vi "HFRR ADV v07 new software.vi"() -> ()   [LabVIEW 2025] (continued)
              n1275 = local write "Language Selection"(w1589) -> ()
            }
            frame 11 {
              n1276 = local write "CH-POWER +"(w1590) -> ()
            }
            frame 12 {
              n1277 = local write "CH-POWER -"(w1591) -> ()
            }
            frame 13 {
              n1278 = local write "CH-HEATER"(w1592) -> ()
            }
            frame 14 {
              n1279 = local write "CH-HUMIDITY WET"(w1593) -> ()
            }
            frame 15 {
              n1280 = local write "CH-HUMIDITY DRY"(w1594) -> ()
            }
            frame 16 {
            }
            frame 17 {
              n1281 = local write "AIR TEMP INTERCEPT:"(w1595) -> ()
            }
            frame 18 {
              n1282 = local write "TEMP INTERCEPT:"(w1596) -> ()
            }
            frame 21 {
              n1283 = local write "S.NO"(w1597) -> ()
            }
            frame 22 {
              n1284 = local write "Com Port 3"(w1598) -> ()
            }
            frame 20 {
              n1285 = local write "Camera Port :"(w1599) -> ()
            }
            frame 19 {
              n1286 = local write "C3 :"(w1600) -> ()
            }
            frame 23, Default {
            }
          }
        }
      }
    }
    n1287 = Select(t=u32 2500 ("milliseconds to wait"), s=w1553, f=u32 500 ("milliseconds to wait")) -> (s? t:f=w1551:u32)
    n1288 = Multiply(x=w1556, y=w1551) -> (x*y=w1558:dbl)
    n1289 = property on="Time slide" class="Slide (strict)"("Visible"=w1547) -> ()  [unwired: 2 in, 2 out]
    n1290 = call "Elapsed Time2"("Time Target (s)"=w1558, "Auto Reset"=TRUE) -> ("Time has Elapsed"=w1548:bool)  [unwired: 10 in, 7 out]
    n1291 = case shown="True" w1548 {
      frame False {
      }
      frame True {
        n1292 = stacked-sequence {
          frame #0 {
            # "DATA PROCESSING"
            # "115 mV/N"
            n1293 = local read "Sample Temperature"() -> (w1601:dbl)
            "TEMP 2" <- w1601
            "TEMP 3" <- w1601
            n1294 = local read "RH Numeric:"() -> (w1608:dbl)
            n1295 = local read "HUMIDITY:"() -> (w1609:dbl)
            n1296 = local read "FRICVALZ"() -> (w1620:dbl)
            n1297 = local read "Friction"() -> (w1604:dbl)
            n1298 = local write "TEMP"(w1601) -> ()
            n1299 = Multiply(x=w1608, y=w1609) -> (x*y=→"Humidity ( %RH )" →"Hum" →"Hum 2":dbl)
            n1300 = Subtract(x=w1604, y=w1620) -> (x-y=w1615:dbl)
            "FF 2" <- w1615
            "FF 4" <- w1615
            n1301 = local read "Ambient Temperature"() -> (→"AIR TEMP":dbl)
            n1302 = local read "TEMP"() -> (w1619:dbl)
            n1303 = local write "FF 3"(w1615) -> ()
            n1304 = Compound Arithmetic op=OR("FRICVALZ 4", "FRICVALZ 3", "FRICVALZ 2") -> (w1611:bool)
            n1305 = case shown="True" w1611 {
              tunnel: w1604 -> [_ w1626]
              frame False {
              }
              frame True {
                w1625 = FALSE ("FRICVALZ")
                n1306 = local write "FRICVALZ 3"(w1625) -> ()
                n1307 = local write "FRICVALZ 2"(w1625) -> ()
                n1308 = local write "FRICVALZ 4"(w1625) -> ()
                "FRICVALZ" <- w1626
              }
            }
            n1309 = Not A Number/Path/Refnum?(number/path/refnum=w1619) -> (NaN/Path/Refnum?=w1618:bool)
            n1310 = Not A Number/Path/Refnum?(number/path/refnum=w1615) -> (NaN/Path/Refnum?=w1617:bool)
            n1311 = Divide(x=w1615, y=1.96) -> (x/y=w1612:dbl)
            n1312 = Compound Arithmetic op=OR(w1618, w1617) -> (w1616:bool)
            n1313 = Not A Number/Path/Refnum?(number/path/refnum=w1612) -> (NaN/Path/Refnum?=w1613:bool)
            n1314 = case shown="True" w1616 {
              frame False {
              }
              frame True {
                n1315 = local write "TEMP"(0.0 ("TEMP")) -> ()
                n1316 = local write "FF 2"(0.0 ("FF 2")) -> ()
                n1317 = local write "reinit"(TRUE ("reinit")) -> ()
              }
            }
            n1318 = Select(t=0.0, s=w1613, f=w1612) -> (s? t:f=w1603:dbl)
            "COF 2" <- w1603
            n1319 = local write "COF 3"(w1603) -> ()
          }
        }
      }
    }
    n1320 = Wait (ms)(milliseconds to wait=u32 50) -> ()  [unwired: 1 out]
    n1321 = local read "Quit"() -> (w1540:bool)
    "Rate" <- 2500.0 ("No of Samples")
  }
  n1322 = while {
    tunnel: w57 -> [_]
    tunnel: [w1653] -> _
    tunnel: [w1629] -> w56
    i -> [w1653]
    stop <- w1629 stop-if-true
    # "C:\\LAB-IQ-NXT\\Scar View.exe"
    n1323 = local read "OK Button 16"() -> (w1642:bool)
    n1324 = local read "Main Tab"() -> (w1635:T2)
    n1325 = local read "service 3"() -> (w1636:bool)
    n1326 = local read "OPEN 6"() -> (w1638:bool)
    n1327 = local read "EDIT 2"() -> (w1640:bool)
    n1328 = flat-sequence {
      frame #0 {
        n1329 = local read "SAVE 2"() -> (w2255:bool)
        n1330 = stacked-sequence {
          frame #0 {
            n1331 = local read "EDIT"() -> (w2309:bool)
            n1332 = case shown="True" w2309 {
              tunnel: [u8 2 ("Disabled") u8 0 ("Disabled")] -> _
              frame False {
                w2311 = FALSE
                n1333 = local write "Password"("") -> ()
                n1334 = property on="SrvM CP" class="Bool (strict)"("Visible"=w2311) -> ()  [unwired: 2 in, 2 out]
                n1335 = property on="message" class="Str"("Visible"=w2311) -> ()  [unwired: 2 in, 2 out]
                n1336 = local write "x = y?"(w2311) -> ()
                n1337 = property on="Password" class="Str"("Visible"=w2311) -> ()  [unwired: 2 in, 2 out]
                n1338 = property on="ENTER THE NEW PASSWORD" class="Str"("Visible"=w2311) -> ()  [unwired: 2 in, 2 out]
                n1339 = property on="ENTER CURRENT PASSWORD" class="Str"("Visible"=w2311) -> ()  [unwired: 2 in, 2 out]
                n1340 = local write "SrvM CP"(w2311) -> ()
              }
              frame True {
                w2314 = TRUE
                n1341 = property on="SrvM CP" class="Bool (strict)"("Visible"=w2314) -> ()  [unwired: 2 in, 2 out]
                n1342 = property on="Password" class="Str"("Visible"=w2314) -> ()  [unwired: 2 in, 2 out]
              }
            }
            "dipl pwd" <- "@143$\n" ("dipl pwd")
          }
          frame #1 {
            # "Gain password"
            n1343 = String To Byte Array(string="ENTER CURRENT PASSWORD") -> (unsigned byte array=w2319:u8[])
            n1344 = Search 1D Array(1D array=w2319, element=u8 10) -> (index of element=w2322:i32)  [unwired: 1 in]
            n1345 = Index Array(array=w2319, index=w2322) -> (element=w2318:u8)
            n1346 = Equal?(x=w2318, y=10) -> (x = y?=w2316:bool)
            n1347 = case shown="True" w2316 {
              frame False {
                n1348 = property on="ENTER THE NEW PASSWORD" class="Str"("Visible"=FALSE) -> ()  [unwired: 2 in, 2 out]
              }
              frame True {
                # "password"
                # "change password logic"
                n1349 = local read "ENTER CURRENT PASSWORD"() -> (w2335:string)
                n1350 = local read "dipl pwd"() -> (w2329:string)
                n1351 = String To Byte Array(string=w2335) -> (unsigned byte array=w2337:u8[])
                n1352 = String To Byte Array(string=w2329) -> (unsigned byte array=w2330:u8[])
                n1353 = Array Size(array=w2337) -> (size(s)=w2334:i32)
                n1354 = Array Size(array=w2330) -> (size(s)=w2332:i32)
                n1355 = for {
                  N: w2334 -> [_]
                  tunnel: w2337 -> [w2361]
                  tunnel: [w2359] -> w2338 mode=indexing
                  tunnel: w2334 -> [w2353]
                  i -> [w2354]
                  n1356 = Decrement(x=w2353) -> (x-1=w2351:i32)
                  n1357 = Equal?(x=w2354, y=w2351) -> (x = y?=w2352:bool)
                  n1358 = Index Array(array=w2361, index=w2354) -> (element=w2355:u8)
                  n1359 = Number To Decimal String(number=w2355) -> (decimal integer string=w2360:string)  [unwired: 1 in]
                  n1360 = Select(t="", s=w2352, f="\r") -> (s? t:f=w2357:string)
                  n1361 = Concatenate Strings(w2360, w2357) -> (w2359:string)
                }
                n1362 = for {
                  N: w2332 -> [_]
                  tunnel: w2330 -> [w2349]
                  tunnel: [w2347] -> w2331 mode=indexing
                  tunnel: w2332 -> [w2344]
                  i -> [w2345]
                  n1363 = Decrement(x=w2344) -> (x-1=w2343:i32)
                  n1364 = Equal?(x=w2345, y=w2343) -> (x = y?=w2342:bool)
                  n1365 = Index Array(array=w2349, index=w2345) -> (element=w2348:u8)
                  n1366 = Number To Decimal String(number=w2348) -> (decimal integer string=w2346:string)  [unwired: 1 in]
                  n1367 = Select(t="", s=w2342, f="\r") -> (s? t:f=w2339:string)
                  n1368 = Concatenate Strings(w2346, w2339) -> (w2347:string)
                }
                n1369 = local read "string"() -> (w2336:string)
                n1370 = Concatenate Strings(w2331) -> (w2325:string)
                n1371 = Concatenate Strings(w2336) -> (w2333:string)
                n1372 = Concatenate Strings(w2338) -> (w2326:string)
                n1373 = Equal?(x=w2326, y=w2333) -> (x = y?=w2328:bool)
                n1374 = Equal?(x=w2326, y=w2325) -> (x = y?=w2324:bool)
                n1375 = Or(x=w2328, y=w2324) -> (x .or. y?=w2327:bool)
                n1376 = case shown="True" w2327 {
                  frame False {
                  }
                  frame True {
                    n1377 = property on="ENTER THE NEW PASSWORD" class="Str"("Visible"=TRUE) -> ()  [unwired: 2 in, 2 out]
                  }
                }
              }
            }
          }
          frame #2 {
            n1378 = String To Byte Array(string="ENTER THE NEW PASSWORD") -> (unsigned byte array=w2364:u8[])
            n1379 = Search 1D Array(1D array=w2364, element=u8 10) -> (index of element=w2368:i32)  [unwired: 1 in]
            n1380 = Index Array(array=w2364, index=w2368) -> (element=w2366:u8)
            n1381 = Equal?(x=w2366, y=10) -> (x = y?=w2363:bool)
            n1382 = case shown="False" w2363 {
              frame False {
              }
              frame True {
                n1383 = local write "EDIT"(FALSE) -> ()
                n1384 = local write "SrvM CP"(FALSE) -> ()
                n1385 = local read "ENTER THE NEW PASSWORD"() -> (w2371:string)
                n1386 = String To Byte Array(string=w2371) -> (unsigned byte array=w2376:u8[])
                n1387 = Array Size(array=w2376) -> (size(s)=w2373:i32)
                n1388 = for {
                  N: w2373 -> [_]
                  tunnel: w2376 -> [w2389]
                  tunnel: [w2386] -> w2378 mode=indexing
                  tunnel: w2373 -> [w2381]
                  i -> [w2379]
                  n1389 = Decrement(x=w2381) -> (x-1=w2382:i32)
                  n1390 = Equal?(x=w2379, y=w2382) -> (x = y?=w2383:bool)
                  n1391 = Index Array(array=w2389, index=w2379) -> (element=w2388:u8)
                  n1392 = Number To Decimal String(number=w2388) -> (decimal integer string=w2387:string)  [unwired: 1 in]
                  n1393 = Select(t="", s=w2383, f="\r") -> (s? t:f=w2380:string)
                  n1394 = Concatenate Strings(w2387, w2380) -> (w2386:string)
                }
                n1395 = local read "file path"() -> (w2370:path)
                n1396 = Concatenate Strings(w2378) -> (w2372:string)
                n1397 = Delete(path (use dialog)=w2370) -> (deleted path=w2374:path)  [unwired: 4 in, 2 out]
                n1398 = call <vilib>:"Write Characters To File.vi"("append to file? (new file:F)"=FALSE, "character string"=w2372, "file path (dialog if empty)"=w2374) -> ()  [unwired: 2 in, 1 out]
              }
            }
          }
          frame #3 {
            n1399 = case shown="True" "SrvM CP" {
              frame False {
                w2392 = ""
                n1400 = local write "ENTER CURRENT PASSWORD"(w2392) -> ()
                n1401 = local write "ENTER THE NEW PASSWORD"(w2392) -> ()
                n1402 = property on="ENTER CURRENT PASSWORD" class="Str"("Visible"=FALSE) -> ()  [unwired: 2 in, 2 out]
              }
              frame True {
                n1403 = property on="ENTER THE NEW PASSWORD" class="Str"() -> ("Visible"=w2393:bool)  [unwired: 2 in, 2 out]
                n1404 = Not(x=w2393) -> (.not. x?=w2394:bool)
                n1405 = property on="ENTER CURRENT PASSWORD" class="Str"("Visible"=w2394) -> ()  [unwired: 2 in, 2 out]
              }
            }
          }
          frame #4 {
            n1406 = String To Byte Array(string="Password") -> (unsigned byte array=w2401:u8[])
            n1407 = Search 1D Array(1D array=w2401, element=u8 10) -> (index of element=w2399:i32)  [unwired: 1 in]
            n1408 = Index Array(array=w2401, index=w2399) -> (element=w2400:u8)
            n1409 = Equal?(x=w2400, y=10) -> (x = y?=w2396:bool)
            n1410 = case shown="True" w2396 {
              frame False {
              }
              frame True {
                # "password"
                # "password"
                n1411 = local read "Password"() -> (w2414:string)
                n1412 = String To Byte Array(string=w2414) -> (unsigned byte array=w2417:u8[])
                n1413 = String To Byte Array(string="@143$\n") -> (unsigned byte array=w2403:u8[])
                n1414 = Array Size(array=w2417) -> (size(s)=w2412:i32)
                n1415 = Array Size(array=w2403) -> (size(s)=w2408:i32)
                n1416 = for {
                  N: w2412 -> [_]
                  tunnel: w2417 -> [w2451]
                  tunnel: [w2449] -> w2418 mode=indexing
                  tunnel: w2412 -> [w2446]
                  i -> [w2447]
                  n1417 = Decrement(x=w2446) -> (x-1=w2445:i32)
                  n1418 = Index Array(array=w2451, index=w2447) -> (element=w2450:u8)
                  n1419 = Equal?(x=w2447, y=w2445) -> (x = y?=w2444:bool)
                  n1420 = Number To Decimal String(number=w2450) -> (decimal integer string=w2448:string)  [unwired: 1 in]
                  n1421 = Select(t="", s=w2444, f="\r") -> (s? t:f=w2441:string)
                  n1422 = Concatenate Strings(w2448, w2441) -> (w2449:string)
                }
                n1423 = for {
                  N: w2408 -> [_]
                  tunnel: w2403 -> [w2462]
                  tunnel: [w2460] -> w2406 mode=indexing
                  tunnel: w2408 -> [w2457]
                  i -> [w2458]
                  n1424 = Decrement(x=w2457) -> (x-1=w2456:i32)
                  n1425 = Index Array(array=w2462, index=w2458) -> (element=w2461:u8)
                  n1426 = Equal?(x=w2458, y=w2456) -> (x = y?=w2455:bool)
                  n1427 = Number To Decimal String(number=w2461) -> (decimal integer string=w2459:string)  [unwired: 1 in]
                  n1428 = Select(t="", s=w2455, f="\r") -> (s? t:f=w2452:string)
                  n1429 = Concatenate Strings(w2459, w2452) -> (w2460:string)
                }
                n1430 = local read "file path"() -> (w2402:path)
                n1431 = call <vilib>:"Read Characters From File.vi"("file path (dialog if empty)"=w2402) -> ("character string"=w2416:string)  [unwired: 5 in, 3 out]
                "string" <- w2416
                n1432 = flat-sequence {
                  tunnel: [w2419] -> w2413
                  frame #0 {
                    w2419 = ""
                    n1433 = local write "Password"(w2419) -> ()
                  }
                }
                n1434 = Concatenate Strings(w2406) -> (w2407:string)
                n1435 = Concatenate Strings(w2416) -> (w2415:string)
                n1436 = Concatenate Strings(w2418) -> (w2410:string)
                n1437 = Equal?(x=w2410, y=w2415) -> (x = y?=w2405:bool)
                n1438 = Equal?(x=w2410, y=w2407) -> (x = y?=w2411:bool)
                n1439 = Or(x=w2405, y=w2411) -> (x .or. y?=w2404:bool)
                "x = y?" <- w2404
                n1440 = case shown="True" w2404 {
                  selector: w2404 -> [w2421 _]
                  tunnel: w2413 -> [_ _]
                  frame False {
                    n1441 = And(x=w2421, y=TRUE ("Visible")) -> (x .and. y?=w2422:bool)
                    n1442 = property on="message" class="Str"("Visible"=w2422) -> ()  [unwired: 2 in, 2 out]
                  }
                  frame True {
                    n1443 = control-ref of="This VI"() -> (w2433:refnum<vi>)
                    n1444 = property class="VI"(reference=w2433) -> (reference out=w2424:refnum<vi>, error out=w2428:errorcluster, "Panel"=w2432:refnum<vi>)  [unwired: 1 in]
                    n1445 = property on="message" class="Str"("Visible"=FALSE) -> ()  [unwired: 2 in, 2 out]
                    n1446 = property class="Pnl"(reference=w2432, error in=w2428) -> (reference out=w2426:refnum<vi>, error out=w2429:errorcluster, "Panes[]"=w2431:refnum<vi>[])
                    n1447 = for {
                      tunnel: w2431 -> [w2440] mode=indexing
                      tunnel: T18."Always On" ("Horizontal Scrollbar Visibility") -> [w2439]
                      tunnel: w2429 -> [w2436]
                      tunnel: [w2435] -> w2427
                      n1448 = property class="Pane"(reference=w2440, error in=w2436, "HorizScrollbarVisibility"=w2439) -> (reference out=w2437:refnum<vi>, error out=w2438:errorcluster)
                      n1449 = Close Reference(reference=w2437, error in (no error)=w2438) -> (error out=w2435:errorcluster)
                    }
                    n1450 = Close Reference(reference=w2426, error in (no error)=w2427) -> (error out=w2425:errorcluster)
                    n1451 = Close Reference(reference=w2424, error in (no error)=w2425) -> (error out=→"error out 6":errorcluster)
                  }
                }
              }
            }
          }
        }
        n1452 = local read "x = y?"() -> (w2261:bool)
        n1453 = local read "HUMIDITY: 2"() -> (w2263:dbl)
        n1454 = local read "HUMIDITY:"() -> (w2262:dbl)
        n1455 = property on="Port 2 Error" class="Clust (strict)"("Visible"="EDIT") -> ()  [unwired: 2 in, 2 out]
        n1456 = property on="Port 1 Error" class="Clust (strict)"("Visible"="EDIT") -> ()  [unwired: 2 in, 2 out]
        n1457 = case shown="True" "SrvM CP 2" {
          frame False {
          }
          frame True {
            n1458 = local write "SrvM CP 2"(FALSE ("SrvM CP 2")) -> ()
            n1459 = local read "HUMIDITY: 2"() -> (w2302:dbl)
            n1460 = local read "TEMP INTERCEPT: 2"() -> (w2301:dbl)
            n1461 = local read "DISPLACEMENT : 4"() -> (w2305:dbl)
            n1462 = local read "TEMPERATURE : 2"() -> (w2304:dbl)
            n1463 = local read "STROKE GAIN : 2"() -> (w2306:dbl)
            n1464 = local read "FRIC. FORCE : 2"() -> (w2307:dbl)
            n1465 = local read "AIR TEMP INTERCEPT: 2"() -> (w2300:dbl)
            n1466 = local read "AIR TEMPERATURE : 2"() -> (w2303:dbl)
            n1467 = local write "HUMIDITY:"(w2302) -> ()
            n1468 = local write "AIR TEMP INTERCEPT:"(w2301) -> ()
            n1469 = local write "TEMPERATURE :"(w2304) -> ()
            n1470 = local write "FRIC. FORCE :"(w2307) -> ()
            n1471 = local write "STROKE GAIN :"(w2306) -> ()
            n1472 = local write "DISPLACEMENT :"(w2305) -> ()
            n1473 = local write "AIR TEMPERATURE :"(w2303) -> ()
            n1474 = local write "TEMP INTERCEPT:"(w2300) -> ()
          }
        }
        n1475 = Or(x="SAVE", y=w2255) -> (x .or. y?=w2256:bool)
        n1476 = And(x="EDIT", y=w2261) -> (x .and. y?=w2259:bool)
        n1477 = local read "DISPLACEMENT : 4"() -> (w2272:dbl)
        n1478 = local read "TEMPERATURE : 2"() -> (w2270:dbl)
        n1479 = local read "STROKE GAIN : 2"() -> (w2276:dbl)
        n1480 = local read "DISPLACEMENT :"() -> (w2271:dbl)
        n1481 = local read "FRIC. FORCE : 2"() -> (w2279:dbl)
        n1482 = local read "TEMPERATURE :"() -> (w2268:dbl)
        n1483 = local read "STROKE GAIN :"() -> (w2275:dbl)
        n1484 = local read "FRIC. FORCE :"() -> (w2278:dbl)
        n1485 = case shown="True" w2259 {
          tunnel: [u8 2 ("Disabled") u8 0 ("Disabled")] -> w2258
          tunnel: [w2623 TRUE ("Visible")] -> w2257
          frame False {
            w2623 = FALSE ("Visible")
            n1486 = local write "EDIT 2"(w2623) -> ()
          }
          frame True {
          }
        }
        n1487 = case shown="True" w2256 {
          frame False {
          }
          frame True {
            n1488 = stacked-sequence {
              seq-local: [w2471 _ _] -> [_ w2618 _]
              frame #0 {
                (unwired) i16 5 ("precision (6)")
                # "[CH1]    - FF\n[CH2]   - TEMPERATURE\n[CH3]    - Humidity\n[CH4]    - AIR TEMP\n[CH5]\\- Visa Uno\n[CH6] \\- Visa Due\n[CH7]  \\- file path\n[CH8]   - Displacement Gain\n[CHA]   - Stroke Gain\n[CHB]   - Stroke PID Gain\n[CHC]   -Language Selection\n[CHD]   -Power +\n[CHE]   -Power_\n[CHF]   -Heater\n[CHG]   -Humidity Wet\n[CHH]   -Humidity Dry\n[CHI]   -Integral Time"
                n1489 = local read "Language Selection"() -> (w2519:enum16{"English", "Russian"})
                n1490 = local read "CH-HUMIDITY WET"() -> (w2477:u16)
                n1491 = local read "CH-HUMIDITY DRY"() -> (w2474:u16)
                n1492 = local read "STROKE GAIN :"() -> (w2463:dbl)
                n1493 = local read "CH-POWER +"() -> (w2486:u16)
                n1494 = local read "CH-POWER -"() -> (w2483:u16)
                n1495 = local read "CH-HEATER"() -> (w2480:u16)
                n1496 = local read "AIR TEMPERATURE :"() -> (w2466:dbl)
                n1497 = local read "DISPLACEMENT :"() -> (w2464:dbl)
                n1498 = local read "TEMPERATURE :"() -> (w2467:dbl)
                n1499 = local read "FRIC. FORCE :"() -> (w2468:dbl)
                n1500 = local read "HUMIDITY:"() -> (w2465:dbl)
                n1501 = Path To String(path="File Path") -> (string=w2535:string)
                n1502 = Number To Fractional String(number=w2463, width (-)=i16 10 ("precision (6)"), precision (6)=i16 5) -> (F-format string=w2526:string)  [unwired: 1 in]
                n1503 = Number To Fractional String(number=w2519, width (-)=i16 10 ("precision (6)"), precision (6)=i16 5) -> (F-format string=w2515:string)  [unwired: 1 in]
                n1504 = Number To Fractional String(number=w2486, width (-)=i16 10 ("precision (6)"), precision (6)=i16 5) -> (F-format string=w2509:string)  [unwired: 1 in]
                n1505 = Number To Fractional String(number=w2483, width (-)=i16 10 ("precision (6)"), precision (6)=i16 5) -> (F-format string=w2506:string)  [unwired: 1 in]
                n1506 = Number To Fractional String(number=w2480, width (-)=i16 10 ("precision (6)"), precision (6)=i16 5) -> (F-format string=w2501:string)  [unwired: 1 in]
                n1507 = Number To Fractional String(number=w2477, width (-)=i16 10 ("precision (6)"), precision (6)=i16 5) -> (F-format string=w2498:string)  [unwired: 1 in]
                n1508 = Number To Fractional String(number=w2474, width (-)=i16 10 ("precision (6)"), precision (6)=i16 5) -> (F-format string=w2493:string)  [unwired: 1 in]
                n1509 = local read "Com Port 1"() -> (w2470:refnum<visa-resource-name>)
                n1510 = local read "Com Port 2"() -> (w2469:refnum<visa-resource-name>)
                n1511 = Concatenate Strings(w2535, "\\" ("string")) -> (w2534:string)
                n1512 = Number To Fractional String(number=w2468, width (-)=i16 10 ("precision (6)"), precision (6)=i16 5) -> (F-format string=w2567:string)  [unwired: 1 in]
                n1513 = Number To Fractional String(number=w2467, width (-)=i16 10 ("precision (6)"), precision (6)=i16 5) -> (F-format string=w2566:string)  [unwired: 1 in]
                n1514 = Number To Fractional String(number=w2465, width (-)=i16 10 ("precision (6)"), precision (6)=i16 5) -> (F-format string=w2560:string)  [unwired: 1 in]
                n1515 = Number To Fractional String(number=w2466, width (-)=i16 10 ("precision (6)"), precision (6)=i16 5) -> (F-format string=w2554:string)  [unwired: 1 in]
                n1516 = Number To Fractional String(number=w2464, width (-)=i16 10 ("precision (6)"), precision (6)=i16 5) -> (F-format string=w2527:string)  [unwired: 1 in]
                n1517 = Concatenate Strings("[CHA]" ("string"), w2526, "- Stroke Gain" ("string"), "\r") -> (w2520:string)
                n1518 = Concatenate Strings("[CHC]" ("string"), w2515, "-Language Selection" ("string"), "\r") -> (w2512:string)
                n1519 = Concatenate Strings("[CHD]" ("string"), w2509, "-Power +" ("string"), "\r") -> (w2491:string)
                n1520 = Concatenate Strings("[CHG]" ("string"), w2498, "-Humidity Wet" ("string"), "\r") -> (w2488:string)
                n1521 = Concatenate Strings("[CHH]" ("string"), w2493, "-Humidity Dry" ("string"), "\r") -> (w2487:string)
                n1522 = Concatenate Strings("[CH1]" ("string"), w2567, " - FF" ("string"), "\r") -> (w2565:string)
                n1523 = Concatenate Strings("[CH2]" ("string"), w2566, " - TEMPERATURE" ("string"), "\r") -> (w2564:string)
                n1524 = Concatenate Strings("[CH3]" ("string"), w2560, " - Humidity" ("string"), "\r") -> (w2557:string)
                n1525 = Concatenate Strings("[CH4]" ("string"), w2554, " - AIR TEMP" ("string"), "\r") -> (w2550:string)
                n1526 = Concatenate Strings("[CH5]" ("string"), w2470, "- Visa Uno" ("string"), "\r") -> (w2543:string)
                n1527 = Concatenate Strings("[CH6]" ("string"), w2469, "- Visa Due" ("string"), "\r") -> (w2538:string)
                n1528 = Concatenate Strings("[CH7]" ("string"), w2534, "- file path" ("string"), "\r") -> (w2537:string)
                n1529 = Concatenate Strings("[CH8]" ("string"), w2527, "- Displacement Gain" ("string"), "\r") -> (w2530:string)
                n1530 = Concatenate Strings("[CHE]" ("string"), w2506, "-Power_" ("string"), "\r") -> (w2490:string)
                n1531 = Concatenate Strings("[CHF]" ("string"), w2501, "-Heater" ("string"), "\r") -> (w2489:string)
                n1532 = Concatenate Strings(w2565, w2564, w2557, w2550, w2543, w2538, w2537, w2530, w2520, w2512, w2491, w2490, w2489, w2488, w2487) -> (w2471:string)
                "gain" <- w2471
              }
              frame #1 {
                n1533 = local read "Camera Port :"() -> (w2579:string)
                n1534 = local read "C3 :"() -> (w2587:refnum<visa-resource-name>)
                n1535 = local read "TEMP INTERCEPT:"() -> (w2588:dbl)
                n1536 = local read "AIR TEMP INTERCEPT:"() -> (w2589:dbl)
                n1537 = local read "Com Port 3"() -> (w2590:refnum<visa-resource-name>)
                n1538 = Concatenate Strings("[CH8]" ("string"), w2579, "- Visa Camera" ("string"), "\r") -> (w2578:string)
                n1539 = Concatenate Strings("[CH7]" ("string"), w2587, "- Visa Humidity" ("string"), "\r") -> (w2583:string)
                n1540 = Number To Fractional String(number=w2588, width (-)=i16 10 ("precision (6)"), precision (6)=i16 5) -> (F-format string=w2606:string)  [unwired: 1 in]
                n1541 = Concatenate Strings("[CHL]" ("string"), w2590, "- Visa humid" ("string"), "\r") -> (w2593:string)
                n1542 = Number To Fractional String(number=w2589, width (-)=i16 10 ("precision (6)"), precision (6)=i16 5) -> (F-format string=w2613:string)  [unwired: 1 in]
                n1543 = Concatenate Strings("[CHK]" ("string"), w2606, "-TEMP INTERCEPT" ("string"), "\r") -> (w2602:string)
                n1544 = Concatenate Strings("[SNO]" ("string"), "S.NO", "-" ("string"), "\r") -> (w2598:string)
                n1545 = Concatenate Strings("[CHJ]" ("string"), w2613, "-AIR TEMP INTERCEPT" ("string"), "\r") -> (w2603:string)
                n1546 = String To Path(string="C:\\LAB-IQ\\calibrate WO 2465.dcf") -> (path=w2591:path)
                n1547 = Concatenate Strings(w2618, w2603, w2602, w2598, w2593, w2583, w2578) -> (w2617:string)
                n1548 = call <vilib>:"Write Characters To File.vi"("append to file? (new file:F)"=FALSE, "character string"=w2617, "file path (dialog if empty)"=w2591) -> ()  [unwired: 2 in, 1 out]
              }
              frame #2 {
                n1549 = local write "Lan flag"(0.0 ("Lan flag")) -> ()
                n1550 = local write "conststatus"(0.0 ("rpm value : 2")) -> ()
                n1551 = local write "SAVE"(FALSE ("OK Button 14")) -> ()
                n1552 = local write "SAVE 2"(FALSE ("SAVE 2")) -> ()
              }
            }
          }
        }
        n1553 = Subtract(x=w2263, y=w2262) -> (x-y=w2264:dbl)
        n1554 = local read "AIR TEMPERATURE : 2"() -> (w2267:dbl)
        n1555 = local read "AIR TEMPERATURE :"() -> (w2266:dbl)
        n1556 = Divide(x=w2264, y=w2262) -> (x/y=w2286:dbl)
        n1557 = Subtract(x=w2279, y=w2278) -> (x-y=w2277:dbl)
        n1558 = Subtract(x=w2270, y=w2268) -> (x-y=w2269:dbl)
        n1559 = Subtract(x=w2276, y=w2275) -> (x-y=w2274:dbl)
        n1560 = Subtract(x=w2272, y=w2271) -> (x-y=w2273:dbl)
        n1561 = Subtract(x=w2267, y=w2266) -> (x-y=w2265:dbl)
        n1562 = Divide(x=w2277, y=w2278) -> (x/y=w2297:dbl)
        n1563 = Divide(x=w2269, y=w2268) -> (x/y=w2290:dbl)
        n1564 = Divide(x=w2274, y=w2275) -> (x/y=w2294:dbl)
        n1565 = Divide(x=w2273, y=w2271) -> (x/y=w2293:dbl)
        n1566 = Multiply(x=w2286, y=100.0) -> (x*y=→"HUMIDITY  Calibration Error":dbl)
        n1567 = Divide(x=w2265, y=w2266) -> (x/y=w2289:dbl)
        n1568 = Multiply(x=w2297, y=100.0) -> (x*y=→"FRIC. FORCE Calibration Error":dbl)
        n1569 = Multiply(x=w2290, y=100.0) -> (x*y=→"TEMPERATURE  Calibration Error":dbl)
        n1570 = Multiply(x=w2294, y=100.0) -> (x*y=→"STROKE Calibration Error":dbl)
        n1571 = Multiply(x=w2293, y=100.0) -> (x*y=→"DISPLACEMENT  Calibration Error":dbl)
        n1572 = property on="EDIT 2" class="Bool (strict)"("Visible"=w2257) -> ()  [unwired: 2 in, 2 out]
        n1573 = property on="SAVE" class="Bool (strict)"("Visible"=w2257) -> ()  [unwired: 2 in, 2 out]
        n1574 = property on="SrvM CP" class="Bool (strict)"("Disabled"=w2258) -> ()  [unwired: 2 in, 2 out]
        n1575 = property on="visa due" class="CmbBox"("Disabled"=w2258) -> ()  [unwired: 2 in, 2 out]
        n1576 = property on="File Path" class="Path"("Disabled"=w2258) -> ()  [unwired: 2 in, 2 out]
        n1577 = Multiply(x=w2289, y=100.0) -> (x*y=→"AIR TEMPERATURE  Calibration Error":dbl)
        n1578 = property on="Language Selection" class="Enum (strict)"("Visible"=w2257) -> ()  [unwired: 2 in, 2 out]
        n1579 = property on="Tab Control 7" class="TabCtl (strict)"("Disabled"=w2258) -> ()  [unwired: 2 in, 2 out]
        n1580 = property on="AIR TEMP INTERCEPT:" class="DigNum (strict)"("Disabled"=w2258) -> ()  [unwired: 2 in, 2 out]
        n1581 = property on="CH-POWER -" class="DigNum (strict)"("Disabled"=w2258) -> ()  [unwired: 2 in, 2 out]
        n1582 = property on="CH-POWER +" class="DigNum (strict)"("Disabled"=w2258) -> ()  [unwired: 2 in, 2 out]
        n1583 = property on="AIR TEMPERATURE :" class="DigNum (strict)"("Disabled"=w2258) -> ()  [unwired: 2 in, 2 out]
        n1584 = property on="STROKE GAIN :" class="DigNum (strict)"("Disabled"=w2258) -> ()  [unwired: 2 in, 2 out]
        n1585 = property on="SPEED OUT:" class="DigNum (strict)"("Disabled"=w2258) -> ()  [unwired: 2 in, 2 out]
        n1586 = property on="CH-HUMIDITY DRY" class="DigNum (strict)"("Disabled"=w2258) -> ()  [unwired: 2 in, 2 out]
        n1587 = property on="HUMIDITY:" class="DigNum (strict)"("Disabled"=w2258) -> ()  [unwired: 2 in, 2 out]
        n1588 = property on="CH-HUMIDITY WET" class="DigNum (strict)"("Disabled"=w2258) -> ()  [unwired: 2 in, 2 out]
        n1589 = property on="TEMPERATURE :" class="DigNum (strict)"("Disabled"=w2258) -> ()  [unwired: 2 in, 2 out]
        n1590 = property on="DISPLACEMENT :" class="DigNum (strict)"("Disabled"=w2258) -> ()  [unwired: 2 in, 2 out]
        n1591 = property on="CH-HEATER" class="DigNum (strict)"("Disabled"=w2258) -> ()  [unwired: 2 in, 2 out]
        n1592 = property on="TEMP INTERCEPT:" class="DigNum (strict)"("Disabled"=w2258) -> ()  [unwired: 2 in, 2 out]
        n1593 = property on="FRIC. FORCE :" class="DigNum (strict)"("Disabled"=w2258) -> ()  [unwired: 2 in, 2 out]
      }
    }
    n1594 = local read "RUN"() -> (w1652:bool)
    n1595 = local read "RUN"() -> (w1650:bool)
    n1596 = disable-structure shown="Disabled" {
      disable-tunnel: [w1667 _] -> w1633
      disable-tunnel: [w1666 _] -> w1631
      frame Disabled {
        n1597 = local read "Temperature before test"() -> (w1660:dbl)
        n1598 = local read "Temperature after test"() -> (w1673:dbl)
        n1599 = case shown="True" "Save Results" {
          frame False {
          }
          frame True {
            w1689 = "\r"
            n1600 = local write "Save Results"(FALSE ("OK Button 5")) -> ()
            n1601 = local read "Temperature before test"() -> (w1727:dbl)
            n1602 = local read "Temperature after test"() -> (w1729:dbl)
            n1603 = local read "Humidity before test"() -> (w1726:dbl)
            n1604 = local read "Humidity after test"() -> (w1728:dbl)
            n1605 = local read "WS1.4"() -> (w1733:dbl)
            n1606 = local read "AVP"() -> (w1731:dbl)
            n1607 = Number To Fractional String(number=w1733, width (-)=i16 6, precision (6)=i16 1) -> (F-format string=w1693:string)  [unwired: 1 in]
            n1608 = local read "MWSD"() -> (w1730:dbl)
            n1609 = local read "String"() -> (w1722:string)
            n1610 = local read "FILE"() -> (w1725:string)
            n1611 = local read "HCF"() -> (w1732:dbl)
            n1612 = Number To Fractional String(number=w1726, width (-)=i16 6, precision (6)=i16 1) -> (F-format string=w1718:string)  [unwired: 1 in]
            n1613 = Number To Fractional String(number=w1727, width (-)=i16 6, precision (6)=i16 1) -> (F-format string=w1715:string)  [unwired: 1 in]
            n1614 = Number To Fractional String(number=w1728, width (-)=i16 6, precision (6)=i16 1) -> (F-format string=w1711:string)  [unwired: 1 in]
            n1615 = Number To Fractional String(number=w1729, width (-)=i16 6, precision (6)=i16 1) -> (F-format string=w1707:string)  [unwired: 1 in]
            n1616 = Number To Fractional String(number=w1731, width (-)=i16 6, precision (6)=i16 3) -> (F-format string=w1700:string)  [unwired: 1 in]
            n1617 = Concatenate Strings(w1722, w1725) -> (w1744:string)
            n1618 = Number To Fractional String(number=w1730, width (-)=i16 6, precision (6)=i16 1) -> (F-format string=w1704:string)  [unwired: 1 in]
            n1619 = Number To Fractional String(number=w1732, width (-)=i16 6, precision (6)=i16 2) -> (F-format string=w1698:string)  [unwired: 1 in]
            n1620 = Concatenate Strings("(" ("string"), w1693, ")Microns" ("string")) -> (w1692:string)
            n1621 = local read "REMARKS"() -> (w1724:string)
            "REMARKS 2" <- w1724
            n1622 = Concatenate Strings("(" ("string"), w1718, " ) % RH," ("string")) -> (w1719:string)
            n1623 = Concatenate Strings(w1698, ")" ("string")) -> (w1696:string)
            n1624 = Concatenate Strings("(" ("string"), w1715, ")  Deg C ," ("string")) -> (w1714:string)
            n1625 = Concatenate Strings("(" ("string"), w1711, " ) % RH," ("string")) -> (w1710:string)
            n1626 = Concatenate Strings("(" ("string"), w1707, ")  Deg C ," ("string")) -> (w1706:string)
            n1627 = Concatenate Strings("(" ("string"), w1704, ")  Microns," ("string")) -> (w1703:string)
            n1628 = Concatenate Strings("(" ("string"), w1700, ")  kPa," ("string")) -> (w1690:string)
            n1629 = Concatenate Strings(w1744, ".dwm" ("Substring")) -> (w1742:string)
            n1630 = String To Path(string=w1742) -> (path=w1741:path)
            n1631 = Concatenate Strings(w1724, w1689, " Humidity before test= " ("Substring"), w1719, w1689, " Temperature before test = " ("Substring"), w1714, w1689, " Humidity after test= " ("Substring"), w1710, w1689, "Temperature after test = " ("Substring"), w1706, w1689, "MSD = " ("Substring"), w1703, w1689, "  AVP = " ("Substring"), w1690, w1689, "  HCF                     =( " ("Substring"), w1696, w1689, " WS1.4                  = " ("Substring"), w1692, w1689) -> (w1688:string)
            "data" <- w1688
            n1632 = call <vilib>:"Write Characters To File.vi"("append to file? (new file:F)"=FALSE, "character string"=w1688, "file path (dialog if empty)"=w1741) -> ()  [unwired: 2 in, 1 out]
            n1633 = Match Pattern(string=w1688, regular expression="!") -> (after substring=→"export":string)  [unwired: 1 in, 3 out]
          }
        }
        n1634 = Add(x=231.864, y=w1660) -> (x+y=w1657:dbl)
        n1635 = Add(x=231.864, y=w1673) -> (x+y=w1670:dbl)
        n1636 = Divide(x=1705.984, y=w1657) -> (x/y=w1658:dbl)
        n1637 = Divide(x=1705.984, y=w1670) -> (x/y=w1671:dbl)
        n1638 = local read "Humidity before test"() -> (w1662:dbl)
        n1639 = local read "Humidity after test"() -> (w1675:dbl)
        n1640 = Subtract(x=8.017352 ("y"), y=w1658) -> (x-y=w1684:dbl)
        n1641 = Subtract(x=8.017352 ("y"), y=w1671) -> (x-y=w1678:dbl)
        n1642 = expression code="10**y"(w1684) -> (w1664:dbl)
        n1643 = expression code="10**y"(w1678) -> (w1677:dbl)
        n1644 = Multiply(x=w1662, y=w1664) -> (x*y=w1663:dbl)
        n1645 = Multiply(x=w1675, y=w1677) -> (x*y=w1676:dbl)
        n1646 = Divide(x=w1663, y=750.0) -> (x/y=w1679:dbl)
        n1647 = Divide(x=w1676, y=750.0) -> (x/y=w1680:dbl)
        n1648 = Add(x=w1679, y=w1680) -> (x+y=w1681:dbl)
        n1649 = Divide(x=w1681, y=2.0) -> (x/y=w1683:dbl)
        n1650 = local write "AVP"(w1683) -> ()
        n1651 = Subtract(x=1.4, y=w1683) -> (x-y=w1666:dbl)
        n1652 = local read "HCF"() -> (w1667:dbl)
      }
      frame Enabled {
      }
    }
    n1653 = case shown="True" "EDIT 3" {
      frame False {
      }
      frame True {
        n1654 = local write "EDIT 3"(FALSE ("EDIT 3")) -> ()
        n1655 = local write "Main Tab"(T2."About" ("Main Tab")) -> ()
      }
    }
    n1656 = case shown="False" w1652 {
      frame False {
        n1657 = local read "stopT"() -> (w2630:bool)
        n1658 = case shown="True" w2630 {
          frame False {
          }
          frame True {
            n1659 = local write "stopT"(FALSE) -> ()
          }
        }
      }
      frame True {
        "stopT" <- TRUE
      }
    }
    n1660 = case shown="False" w1650 {
      frame False {
      }
      frame True {
      }
    }
    n1661 = case shown="True" w1640 {
      frame False {
        n1662 = property on="Password 2" class="Str"("Visible"=FALSE) -> ()  [unwired: 2 in, 2 out]
        n1663 = local write "Password 2"("" ("Password")) -> ()
      }
      frame True {
        n1664 = property on="Password 2" class="Str"("Visible"=TRUE) -> ()  [unwired: 2 in, 2 out]
        n1665 = Equal?(x="Password 2", y="HFRR1234") -> (x = y?=w1772:bool)
        n1666 = case shown="True" w1772 {
          tunnel: "Password 2" -> [w1775 _]
          frame False {
            n1667 = String Length(string=w1775) -> (length=w1776:i32)
            n1668 = Greater Than 0?(x=w1776) -> (x > 0?=w1774:bool)
            n1669 = case shown="False" w1774 {
              frame False {
                n1670 = property on="Password 2" class="Str"("Caption.Text"="Password (Advance Setting)") -> ()  [unwired: 2 in, 2 out]
              }
              frame True {
                n1671 = property on="Password 2" class="Str"("Caption.Text"="Incorrect Password!") -> ()  [unwired: 2 in, 2 out]
              }
            }
          }
          frame True {
            n1672 = local write "EDIT 2"(FALSE ("EDIT 2")) -> ()
            n1673 = local write "Password 2"("" ("Password")) -> ()
            n1674 = local write "Main Tab"(T2."Advance" ("Main Tab")) -> ()
            n1675 = local write "Main Dashboard Buttons"(T1."Advance" ("Main Dashboard Buttons")) -> ()
          }
        }
      }
    }
    n1676 = case shown="True" "Prog Uno" {
      frame False {
      }
      frame True {
        n1677 = stacked-sequence {
          frame #0 {
            n1678 = Delete(path (use dialog)=path "C:/LAB-IQ-NXT/UNOCOMPILE.bat" ("working directory")) -> ()  [unwired: 4 in, 3 out]
          }
          frame #1 {
            n1679 = local read "Com Port 1"() -> (w2237:refnum<visa-resource-name>)
            n1680 = Concatenate Strings("cmd.exe /c \"mode " ("command line"), w2237, ":1200,n,8,1\"\n" ("command line")) -> (w2242:string)
            n1681 = Concatenate Strings(w2242, "CD\\\nCD WinDucom\navrdude -C avrdude.conf -v -patmega328p -carduino -P" ("command line"), w2237, " -b115200 -D -Uflash:w:UNO_V20.hex:i\n" ("command line"), "\r") -> (w2244:string)
            "STR" <- w2244
            n1682 = call <vilib>:"Write Characters To File.vi"("append to file? (new file:F)"=FALSE, "character string"=w2244, "file path (dialog if empty)"=path "C:/LAB-IQ/UNOCOMPILE.bat" ("working directory")) -> ()  [unwired: 2 in, 1 out]
          }
          frame #2 {
            n1683 = disable-structure shown="Disabled" {
              frame Disabled {
                w2248 = "cmd.exe  /c \"C:\\LAB-IQ-NXT\\UNOCOMPILE.bat\"" ("string")
                n1684 = local write "Prog Uno"(FALSE ("run minimized? (F)")) -> ()
                n1685 = call <vilib>:"System Exec.vi"("expected output size  (4096)"=u32 65535, "run minimized? (F)"=FALSE, "wait until completion? (T)"=TRUE ("run minimized? (F)"), "working directory"=path "C:/LAB-IQ-NXT", "standard input"=w2248, "command line"=w2248) -> ("error out"=w2247:errorcluster, "standard output"=→"String 42":string)  [unwired: 2 in, 2 out]
                "error out 3" <- w2247
                n1686 = flat-sequence {
                  tunnel: w2247 -> [_]
                  frame #0 {
                  }
                }
              }
              frame Enabled {
              }
            }
          }
        }
      }
    }
    n1687 = case shown="\"ISO 12156\"" "TEST STANDARD" {
      tunnel: [2.0 ("Set Temp") 0.0 ("Set Temp") 2.0 ("Set Temp") 0.0 ("Set Temp")] -> w1641
      frame "ASTM D6079", Default {
        w2194 = 50.0 ("Hz")
        w2195 = 53.0 ("Set Rh")
        w2197 = 1.0 ("Set Strk")
        w2196 = 60.0 ("Set Temp")
        # "astm hide"
        n1688 = local write "NORMAL LOAD"(200.0 ("NORMAL LOAD")) -> ()
        n1689 = local write "Set Strk"(w2197) -> ()
        n1690 = local write "Set Hz"(w2194) -> ()
        n1691 = local write "Set Temp"(w2196) -> ()
        n1692 = local write "Set Rh"(w2195) -> ()
        n1693 = local write "test time"(75.0 ("test time")) -> ()
        n1694 = local write "Set Stroke:"(w2197) -> ()
        n1695 = local write "Set Humidity:"(w2195) -> ()
        n1696 = local write "Set Frequency:"(w2194) -> ()
        n1697 = local write "Set Temperature:"(w2196) -> ()
        "Test Standard" <- "ASTM D6079" ("Test Standard 2")
      }
      frame "ISO 12156" {
        n1698 = local write "Set Strk"(1.0 ("Set Strk")) -> ()
        n1699 = local write "NORMAL LOAD"(200.0 ("NORMAL LOAD")) -> ()
        n1700 = local write "Set Temp"(60.0 ("Set Temp")) -> ()
        n1701 = local write "test time"(75.0 ("test time")) -> ()
        n1702 = local write "Set Hz"(50.0 ("Hz")) -> ()
        n1703 = local write "Set Rh"(53.0 ("Set Rh")) -> ()
      }
      frame "CEC F-096-A-06" {
        n1704 = local write "Set Strk"(1.0 ("Set Strk")) -> ()
        n1705 = local write "NORMAL LOAD"(200.0 ("NORMAL LOAD")) -> ()
        n1706 = local write "Set Temp"(60.0 ("Set Temp")) -> ()
        n1707 = local write "test time"(75.0 ("test time")) -> ()
        n1708 = local write "Set Hz"(50.0 ("Hz")) -> ()
        n1709 = local write "Set Rh"(53.0 ("Set Rh")) -> ()
      }
      frame "Custom" {
      }
    }
    n1710 = case shown="True" "Prog Due" {
      frame False {
      }
      frame True {
        n1711 = stacked-sequence {
          frame #0 {
            n1712 = Delete(path (use dialog)=path "C:/LAB-IQ/DUECOMPILE.bat" ("working directory")) -> ()  [unwired: 4 in, 3 out]
          }
          frame #1 {
            n1713 = disable-structure shown="Disabled" {
              frame Disabled {
                n1714 = local read "visa due"() -> (w2219:string)
                n1715 = Concatenate Strings("cmd.exe /c \"mode " ("command line"), w2219, ":1200,n,8,1\"\n" ("command line")) -> (w2224:string)
                n1716 = Concatenate Strings(w2224, "CD\\\nCD WinDucom\nTIMEOUT 1\n bossac.exe -i -d --port=" ("command line"), w2219, " -U false -e -w -v -b DUE.bin -R\n" ("command line"), "\r") -> (w2226:string)
                "concatenated string 2" <- w2226
                n1717 = call <vilib>:"Write Characters To File.vi"("append to file? (new file:F)"=FALSE, "character string"=w2226, "file path (dialog if empty)"=path "C:/LAB-IQ-NXT/DUECOMPILE.bat" ("working directory")) -> ()  [unwired: 2 in, 1 out]
              }
              frame Enabled {
              }
            }
          }
          frame #2 {
            # "C:\\LAB-IQ-NXT\\DUECOMPILE.bat"
            n1718 = disable-structure shown="Disabled" {
              frame Disabled {
                w2231 = "cmd.exe  /c \"C:\\LAB-IQ-NXT\\DUECOMPILE.bat\"" ("string")
                n1719 = call <vilib>:"System Exec.vi"("expected output size  (4096)"=u32 65535, "run minimized? (F)"=FALSE, "wait until completion? (T)"=TRUE ("run minimized? (F)"), "working directory"=path "C:/LAB-IQ-NXT", "standard input"=w2231, "command line"=w2231) -> ("error out"=w2230:errorcluster, "standard output"=→"String 44":string)  [unwired: 2 in, 2 out]
                "error out 4" <- w2230
                n1720 = flat-sequence {
                  tunnel: w2230 -> [_]
                  frame #0 {
                  }
                }
              }
              frame Enabled {
              }
            }
            n1721 = local write "Prog Due"(FALSE ("Prog Due")) -> ()
          }
        }
      }
    }
    n1722 = Or(x=w1638, y=w1636) -> (x .or. y?=w1637:bool)
    n1723 = case shown="\"About\"" w1635 {
      tunnel: [T24."Acquire" ("Main Tab") T24."Compare Files" ("Main Tab") T24."About" ("Main Tab")] -> w1648
      frame "Acquire", Default {
      }
      frame "Compare Files" {
      }
      frame "About" {
      }
    }
    n1724 = Or(x=w1642, y="OPEN") -> (x .or. y?=w1643:bool)
    n1725 = case shown="True" w1643 {
      tunnel: w1642 -> [_ w1783]
      frame False {
      }
      frame True {
        n1726 = stacked-sequence {
          tunnel: w1783 -> [_ w1850 _ _]
          frame #0 {
            w1799 = "  " ("String 6")
            n1727 = local write "OPEN"(FALSE ("open")) -> ()
            n1728 = local read "string1 2"() -> (w1787:string)
            n1729 = local read "string1 3"() -> (w1786:string)
            n1730 = local read "string1 4"() -> (w1785:string)
            n1731 = property on="OPEN" class="Bool (strict)"("Visible"=FALSE) -> ()  [unwired: 2 in, 2 out]
            n1732 = local write "String 6"(w1799) -> ()
            n1733 = local write "String 7"(w1799) -> ()
            n1734 = local write "String 8"(w1799) -> ()
            n1735 = local write "String 12"(w1799) -> ()
            n1736 = local read "OK Button 16"() -> (w1784:bool)
            n1737 = String To Path(string=w1787) -> (path=w1795:path)
            n1738 = String To Path(string=w1786) -> (path=w1794:path)
            n1739 = String To Path(string=w1785) -> (path=w1793:path)
            n1740 = case shown="True" w1784 {
              tunnel: [w1800 w1801] -> w1788
              frame False {
                n1741 = local read "string1"() -> (w1800:string)
              }
              frame True {
                n1742 = local read "String Indicator 4"() -> (w1801:string)
              }
            }
            n1743 = Open/Create/Replace File "Open File"(file path (use dialog)=w1795) -> (refnum out=w1791:refnum<file>)  [unwired: 5 in, 2 out]
            n1744 = Open/Create/Replace File "Open File"(file path (use dialog)=w1794) -> (refnum out=w1790:refnum<file>)  [unwired: 5 in, 2 out]
            n1745 = Open/Create/Replace File "Open File"(file path (use dialog)=w1793) -> (refnum out=w1789:refnum<file>)  [unwired: 5 in, 2 out]
            n1746 = while {
              tunnel: w1791 -> [w1813]
              i -> [w1809]
              stop <- w1808 continue-if-true
              (unwired) TRUE ("line mode (F)")
              n1747 = Read from Text File "Read File"(file (use dialog)=w1813) -> (text=w1810:string)  [unwired: 3 in, 3 out]
              n1748 = local write "Numeric 11"(w1809) -> ()
              n1749 = String Length(string=w1810) -> (length=w1812:i32)
              n1750 = Greater?(x=w1812, y=1) -> (0:w1808:bool)
            }
            n1751 = while {
              tunnel: w1790 -> [w1819]
              i -> [w1815]
              stop <- w1814 continue-if-true
              (unwired) TRUE ("line mode (F)")
              n1752 = Read from Text File "Read File"(file (use dialog)=w1819) -> (text=w1816:string)  [unwired: 3 in, 3 out]
              n1753 = local write "Numeric 12"(w1815) -> ()
              n1754 = String Length(string=w1816) -> (length=w1818:i32)
              n1755 = Greater?(x=w1818, y=1) -> (0:w1814:bool)
            }
            n1756 = while {
              tunnel: w1789 -> [w1825]
              i -> [w1821]
              stop <- w1820 continue-if-true
              (unwired) TRUE ("line mode (F)")
              n1757 = Read from Text File "Read File"(file (use dialog)=w1825) -> (text=w1822:string)  [unwired: 3 in, 3 out]
              n1758 = local write "Numeric 13"(w1821) -> ()
              n1759 = String Length(string=w1822) -> (length=w1824:i32)
              n1760 = Greater?(x=w1824, y=1) -> (0:w1820:bool)
            }
            n1761 = String To Path(string=w1788) -> (path=w1796:path)
            n1762 = Open/Create/Replace File "Open File"(file path (use dialog)=w1796) -> (refnum out=w1792:refnum<file>)  [unwired: 5 in, 2 out]
            n1763 = while {
              tunnel: w1792 -> [w1807]
              i -> [w1803]
              stop <- w1802 continue-if-true
              (unwired) TRUE ("line mode (F)")
              n1764 = Read from Text File "Read File"(file (use dialog)=w1807) -> (text=w1804:string)  [unwired: 3 in, 3 out]
              n1765 = local write "Numeric 8"(w1803) -> ()
              n1766 = String Length(string=w1804) -> (length=w1806:i32)
              n1767 = Greater?(x=w1806, y=1) -> (0:w1802:bool)
            }
          }
          frame #1 {
            w1977 = FALSE ("ACTUAL   MERGE")
            # "Sample Temp"
            # "ECR"
            # "COF"
            # "Time\nCOF\nFF\nTemp"
            n1768 = case shown="True" w1850 {
              tunnel: [w1997 w1998] -> w1851
              frame False {
                n1769 = local read "string1"() -> (w1997:string)
              }
              frame True {
                n1770 = local read "String Indicator 4"() -> (w1998:string)
              }
            }
            n1771 = local read "string1 3"() -> (w1895:string)
            n1772 = String To Path(string=w1851) -> (path=w1982:path)
            n1773 = String To Path(string=w1895) -> (path=w1993:path)
            n1774 = local read "Numeric 12"() -> (w1979:i32)
            n1775 = local read "Numeric 8"() -> (w1981:i32)
            n1776 = local read "string1 2"() -> (w1896:string)
            n1777 = local read "string1 4"() -> (w1894:string)
            n1778 = Open/Create/Replace File "Open File"(file path (use dialog)=w1982) -> (refnum out=w1996:refnum<file>, error out=w1995:errorcluster)  [unwired: 5 in, 1 out]
            n1779 = Open/Create/Replace File "Open File"(file path (use dialog)=w1993) -> (refnum out=w1989:refnum<file>, error out=w1990:errorcluster)  [unwired: 5 in, 1 out]
            n1780 = for {
              N: w1981 -> [_]
              tunnel: w1996 -> [w2144]
              tunnel: w1995 -> [w2143]
              tunnel: [w2133] -> w1908 mode=indexing
              tunnel: [w2131] -> w1965 mode=indexing
              tunnel: [w2132] -> w1960 mode=indexing
              tunnel: w1977 -> [_]
              tunnel: [w2125] -> w1962 mode=indexing
              tunnel: [w2121] -> w1931 mode=indexing
              tunnel: [w2117] -> w1906 mode=indexing
              tunnel: [w2113] -> w1887 mode=indexing
              tunnel: [w2108] -> w1847 mode=indexing
              (unwired) TRUE ("line mode (F)")
              # "freq"
              # "Stroke"
              # "Time"
              # "CoF"
              # "Humidity"
              # "Temp"
              # "Air Temp"
              # "ECR"
              n1781 = Read from Text File "Read File"(file (use dialog)=w2144, error in=w2143) -> (text=w2109:string)  [unwired: 2 in, 3 out]
              n1782 = local write "String 6"(w2109) -> ()
              n1783 = String Subset(string=w2109, offset (0)=0, length (rest)=14 ("length (rest)")) -> (substring=w2137:string)
              n1784 = String Subset(string=w2109, offset (0)=35, length (rest)=9 ("length (rest)")) -> (substring=w2134:string)
              n1785 = String Subset(string=w2109, offset (0)=15, length (rest)=9 ("length (rest)")) -> (substring=w2140:string)
              n1786 = Fract/Exp String To Number(string=w2137) -> (number=w2133:dbl)  [unwired: 3 in, 1 out]
              n1787 = Fract/Exp String To Number(string=w2134) -> (number=w2132:dbl)  [unwired: 3 in, 1 out]
              n1788 = Fract/Exp String To Number(string=w2140) -> (number=w2131:dbl)  [unwired: 3 in, 1 out]
              n1789 = String Subset(string=w2109, offset (0)=85, length (rest)=9 ("length (rest)")) -> (substring=w2110:string)
              n1790 = String Subset(string=w2109, offset (0)=25, length (rest)=9 ("length (rest)")) -> (substring=w2116:string)
              n1791 = String Subset(string=w2109, offset (0)=55, length (rest)=9 ("length (rest)")) -> (substring=w2118:string)
              n1792 = String Subset(string=w2109, offset (0)=45, length (rest)=9 ("length (rest)")) -> (substring=w2124:string)
              n1793 = String Subset(string=w2109, offset (0)=65, length (rest)=9 ("length (rest)")) -> (substring=w2130:string)
              n1794 = Fract/Exp String To Number(string=w2116) -> (number=w2113:dbl)  [unwired: 3 in, 1 out]
              n1795 = Fract/Exp String To Number(string=w2110) -> (number=w2108:dbl)  [unwired: 3 in, 1 out]
              n1796 = Fract/Exp String To Number(string=w2118) -> (number=w2117:dbl)  [unwired: 3 in, 1 out]
              n1797 = Fract/Exp String To Number(string=w2124) -> (number=w2121:dbl)  [unwired: 3 in, 1 out]
              n1798 = Fract/Exp String To Number(string=w2130) -> (number=w2127:dbl)  [unwired: 3 in, 1 out]
              n1799 = Add(x=w2127, y=0.0) -> (x+y=w2125:dbl)
            }
            n1800 = for {
              N: w1979 -> [_]
              tunnel: w1990 -> [w2070]
              tunnel: w1989 -> [w2069]
              tunnel: [w2059] -> w1948 mode=indexing
              tunnel: [w2057] -> w1946 mode=indexing
              tunnel: [w2058] -> w1942 mode=indexing
              tunnel: w1977 -> [_]
              tunnel: [w2051] -> w1944 mode=indexing
              tunnel: [w2047] -> w1926 mode=indexing
              tunnel: [w2043] -> w1902 mode=indexing
              tunnel: [w2040] -> w1883 mode=indexing
              tunnel: [w2036] -> w1842 mode=indexing
              (unwired) 9 ("length (rest)")
              (unwired) 9 ("length (rest)")
              (unwired) TRUE ("line mode (F)")
              n1801 = Read from Text File "Read File"(file (use dialog)=w2069, error in=w2070) -> (text=w2037:string)  [unwired: 2 in, 3 out]
              n1802 = local write "String 8"(w2037) -> ()
